vi "get_visa.vi"(8 "error in (no error)":errorcluster, 11 "SignalWriterMH110203USBStepperMotor in":refnum<class "SignalWriterMH110203USBStepperMotor.lvclass">) -> (0 "error out":errorcluster, 1 "axis":i32, 2 "visa array":refnum<visa-resource-name>[](array[refnum]), 3 "SignalWriterMH110203USBStepperMotor out":refnum<class "SignalWriterMH110203USBStepperMotor.lvclass">)   [LabVIEW 2010, in "SignalWriterMH110203USBStepperMotor.lvclass"]
uses:
  SignalWriterMH110203USBStepperMotor.lvclass
  SignalWriterMH110203USBStepperMotor.lvclass/SignalWriterMH110203USBStepperMotor.ctl
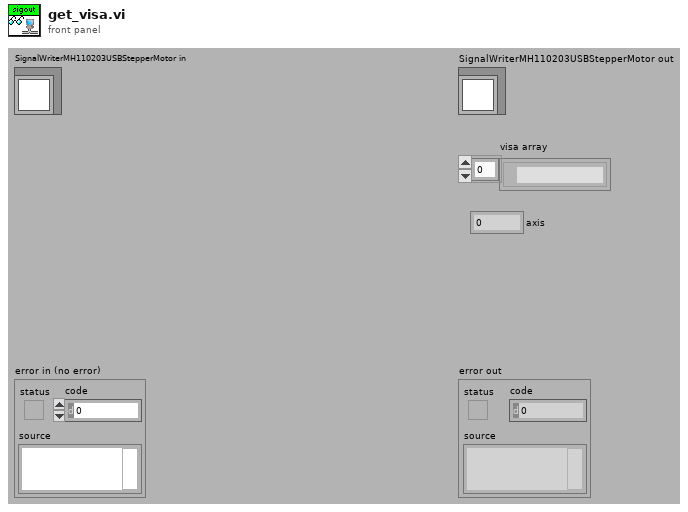
[diagram p1: front panel]
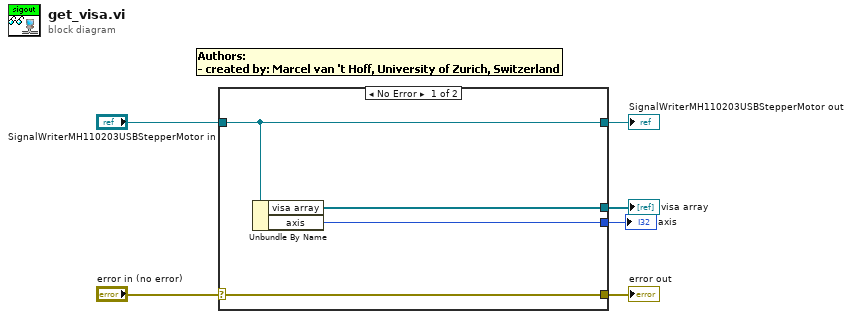
[diagram p0: block diagram]
diagram:
  n1 = case shown="No Error" "error in (no error)" {
    selector: "error in (no error)" -> [w10 w11]
    tunnel: [w10 w11] -> w5
    tunnel: [w9 w12] -> w3
    tunnel: "SignalWriterMH110203USBStepperMotor in" -> [w9 w12]
    tunnel: [w8 _] -> w2
    tunnel: [w7 _] -> w1
    frame No Error {
      n2 = Unbundle By Name(w9) -> ("visa array"=w8:refnum<visa-resource-name>[], "axis"=w7:i32)
    }
    frame Error {
    }
  }
  "error out" <- w5
  "SignalWriterMH110203USBStepperMotor out" <- w3
  "visa array" <- w2
  "axis" <- w1
